vi "AxisConfiguration.vi"(1 "AxisNo":u16) -> (0 "AxisConfigurationOUT":T1={"AxisHomeType"=1, "AxisBacklash"=0.0, "AxisGain"=1.0, "AxisOffset"=0.0, "AxisUnit"=0, "ReqConfRead"=FALSE, "ReqConfWrite"=FALSE, "AxisName"="", "AxisAccDecc"=0.0, "AxisHomeVel"=0.0} {"AxisUnit" items=["mm", "°"]; "AxisHomeType" items=["no homing"=0, "forward limit switch"=1, "backward limit switch"=2, "forward reference"=4, "backward reference"=8]})   [LabVIEW 2020, in "SMCD14_lib.lvlib"]
uses:
  AxisConfiguration_typedef.ctl
  Globals.vi
  SMCD14_lib.lvlib
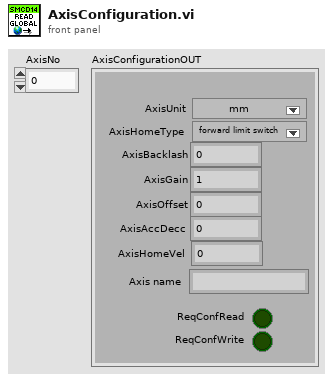
[diagram p1: front panel]
types:
  T1 = typedef "SMCD14_lib.lvlib/AxisConfiguration_typedef.ctl" = cluster{"AxisHomeType":u16, "AxisBacklash":dbl, "AxisGain":dbl, "AxisOffset":dbl, "AxisUnit":u16, "ReqConfRead":bool, "ReqConfWrite":bool, "AxisName":string, "AxisAccDecc":dbl, "AxisHomeVel":dbl}
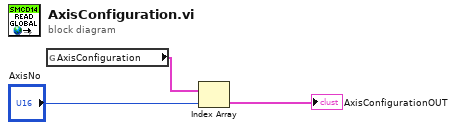
[diagram p0: block diagram]
diagram:
  n1 = global read "Globals.vi" "AxisConfiguration"() -> (w1:T1[])
  n2 = Index Array(array=w1, index="AxisNo") -> (element=→"AxisConfigurationOUT":T1)
